vi "Terminals Descending Order.vi"(10 "Terminals":T1) -> (2 "Terminals Descending Order":i32[](array[numeric]))   [LabVIEW 2025, in "_Rescript.lvlib"]
uses:
  _Rescript.lvlib
  Terminals.ctl
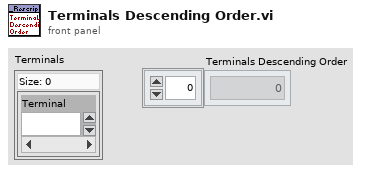
[diagram p1: front panel]
types:
  T1 = typedef "_Rescript.lvlib/Terminals.ctl" = set{i32}
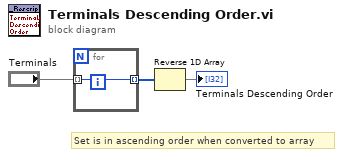
[diagram p0: block diagram]
diagram:
  # "Set is in ascending order when converted to array"
  n1 = for {
    tunnel: "Terminals" -> [w4] mode=indexing
    tunnel: [w4] -> w2 mode=indexing
  }
  n2 = Reverse 1D Array(array=w2) -> (reversed array=→"Terminals Descending Order":i32[])
